vi "Configure CAN Signal.vi"(7 "Signal Type (3: DIFL)":i32(ring)=3 items=["CANH", "CANL", "DIfferential", "DIFL"], 8 "error in (no error)":errorcluster, 9 "Baud Rate (10000 b/s)":dbl=10000.0, 10 "CAN Channel (1: Channel 1)":i32(ring)=1 items=["Channel 1"=1, "Channel 2"=2, "Channel 3"=3, "Channel 4"=4], 11 "VISA resource name":refnum<visa-resource-name>) -> (0 "error out":errorcluster, 3 "VISA resource name out":refnum<visa-resource-name>)   [LabVIEW 2013, in "Agilent 90000 Series.lvlib"]
doc: "Configures the baud rate, and type of the CAN signal.\n\n<b>Notes:</b> \n1. This VI is new in firmware version 4.60.\n2. The signal type can be set when the CAN Trigger is set ti SOF."
uses:
  Agilent 90000 Series.lvlib
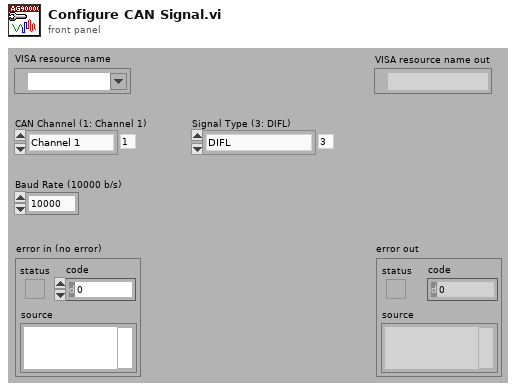
[diagram p1: front panel]
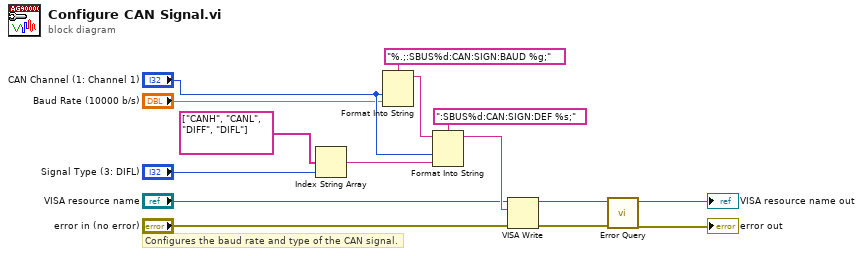
[diagram p0: block diagram]
diagram:
  # "Configures the baud rate and type of the CAN signal."
  n1 = Index String Array(1:"Signal Type (3: DIFL)", 2:string[] ["CANH", "CANL", "DIFF", "DIFL"] ("string array")) -> (0:w2:string)  [unwired: 1 in]
  n2 = Format Into String(format string="%.;:SBUS%d:CAN:SIGN:BAUD %g;", "CAN Channel (1: Channel 1)", "Baud Rate (10000 b/s)") -> (resulting string=w12:string)  [unwired: 2 in, 1 out]
  n3 = Format Into String(format string=":SBUS%d:CAN:SIGN:DEF %s;", initial string=w12, "CAN Channel (1: Channel 1)", w2) -> (resulting string=w10:string)  [unwired: 1 in, 1 out]
  n4 = VISA Write(VISA resource name="VISA resource name", write buffer=w10, error in (no error)="error in (no error)") -> (VISA resource name out=w7:refnum<visa-resource-name>, error out=w6:errorcluster)  [unwired: 1 out]
  n5 = call "Error Query.vi"("error in (no error)"=w6, "VISA resource name"=w7) -> ("error out"=→"error out":errorcluster, "VISA resource name out"=→"VISA resource name out":refnum<visa-resource-name>)  [unwired: 6 in, 2 out]
